vi "List Keys.vi"(8 "error in (no error)":errorcluster, 11 "Variant in":variant) -> (0 "error out":errorcluster, 1 "Values":variant[](array[variant]), 2 "Keys":string[](array[string]), 3 "Variant out":variant)   [LabVIEW 2019, in "JSON.lvlib"]
doc: "Lists the keys and values of the next nested object. Use this VI to traverse the <b>Variant in</b>.\n\nCreated by: Ryan Pacini"
uses:
  JSON.lvlib
  <vilib>/Utility/Data Type/NI_Data Type.lvlib
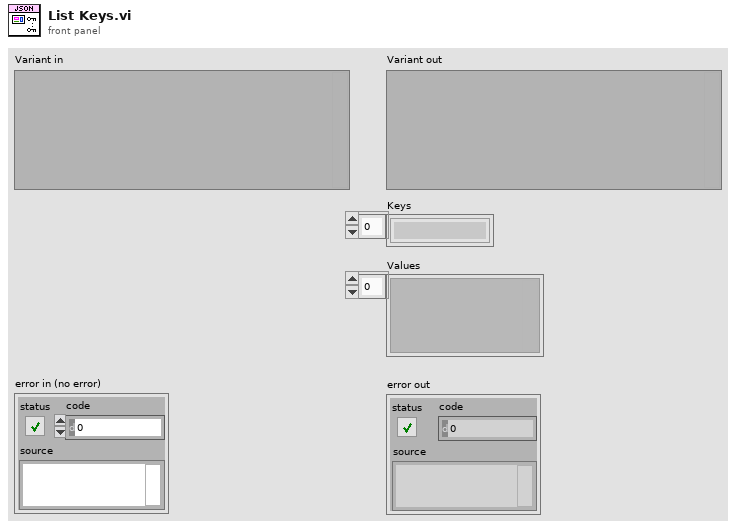
[diagram p1: front panel]
types:
  T1 = typedef "NI_Data Type.lvlib/Data Type.ctl" = enum8{"Invalid Type", "Void", "I8", "I16", "I32", "I64", "U8", "U16", "U32", "U64", "Single Float", "Double Float", "Extended Float", "Single Complex", "Double Complex", "Extended Complex", "Enum U8", "Enum U16", "Enum U32", "Enum U64", "Single Float With Unit", "Double Float With Unit", "Extended Float With Unit", "Single Complex with Unit", "Double Complex with Unit", "Extended Complex with Unit", "Boolean", "String", "Path", "Picture", "Tag", "Array", "Cluster", "Variant", "LV Variant", "Waveform", "Timestamp", "Digital Waveform", "Digital Data", "ExpressData", "Refnum", "External Data", "VI", "Poly VI", "LabVIEW Class Instance", "Fixed Point", "Set Collection", "Map Collection"}
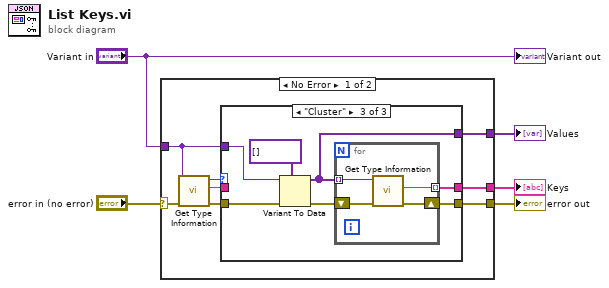
[diagram p0: block diagram]
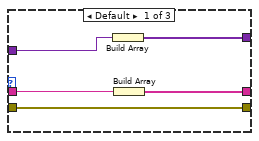
[diagram p2: hidden frame]
diagram:
  n1 = case shown="No Error" "error in (no error)" {
    selector: "error in (no error)" -> [w13 w31]
    tunnel: [w11 w31] -> w4
    tunnel: "Variant in" -> [w10 _]
    tunnel: [w7 _] -> w2
    tunnel: [w6 _] -> w1
    frame No Error {
      n2 = call <vilib>:"Get Type Information.vi"("error in (no error)"=w13, "variant"=w10) -> ("error out"=w12:errorcluster, "name"=w8:string, "type"=w9:T1)  [unwired: 5 in, 2 out]
      n3 = case shown="\"Cluster\"" w9 {
        tunnel: w12 -> [w16 w19 w26]
        tunnel: [w16 w19 w22] -> w11
        tunnel: w10 -> [w15 _ w24]
        tunnel: w8 -> [w18 _ _]
        tunnel: [w17 _ w21] -> w6
        tunnel: [w14 _ w20] -> w7
        frame Default {
          n4 = Build Array(w15) -> (w14:variant[])
          n5 = Build Array(w18) -> (w17:string[])
        }
        frame "Invalid Type", "Void" {
        }
        frame "Cluster" {
          n6 = Variant To Data(error in=w26, type=variant[] [], Variant=w24) -> (data=w20:variant[], error out=w23:errorcluster)
          n7 = for {
            tunnel: w20 -> [w29] mode=indexing
            shift-right: [w28] -> w22
            shift-left: w23 -> [w30]
            tunnel: [w27] -> w21 mode=indexing
            n8 = call <vilib>:"Get Type Information.vi"("error in (no error)"=w30, "variant"=w29) -> ("error out"=w28:errorcluster, "name"=w27:string)  [unwired: 5 in, 3 out]
          }
        }
      }
    }
    frame Error {
    }
  }
  "error out" <- w4
  "Keys" <- w1
  "Values" <- w2
  "Variant out" <- "Variant in"
